vi "GF_SaveAgilentDataBinary.vi"(1 "Array":waveform(dbl)[][](array[waveform]), 2 "Base Path":path) -> (0 "File Write Errors":errorcluster[](array[cluster]))   [LabVIEW 2009]
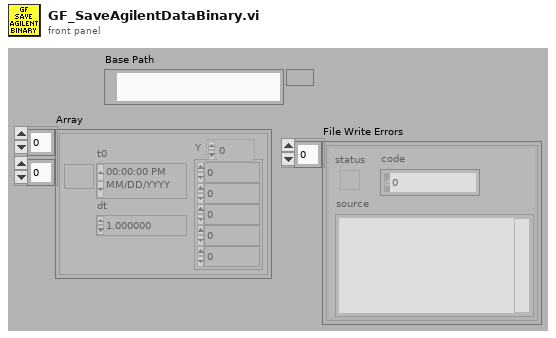
[diagram p1: front panel]
types:
  T1 = enum16{"big-endian, network order", "native, host order", "little-endian"}
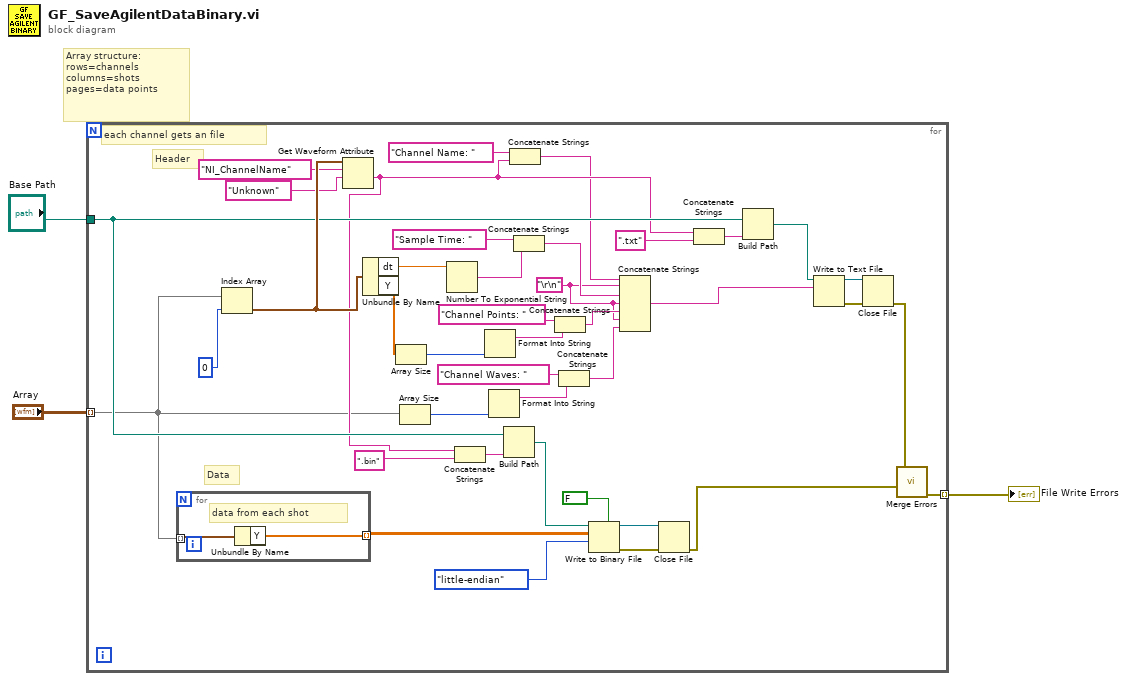
[diagram p0: block diagram]
diagram:
  # "Array structure:\nrows=channels\ncolumns=shots\npages=data points"
  n1 = for {
    tunnel: "Array" -> [w7] mode=indexing
    tunnel: "Base Path" -> [w26]
    tunnel: [w24] -> w1 mode=indexing
    w5 = "\r\n"
    # "Data"
    # "Header"
    # "each channel gets an file"
    n2 = for {
      tunnel: w7 -> [w45] mode=indexing
      tunnel: [w44] -> w31 mode=indexing
      # "data from each shot"
      n3 = Unbundle By Name(w45) -> ("Y"=w44:dbl[])
    }
    n4 = Index Array(array=w7, index=0) -> (element=w42:waveform(dbl))
    n5 = Get Waveform Attribute(5:"Unknown" ("name"), 6:"NI_ChannelName" ("name"), 7:w42) -> (1:w23:string)  [unwired: 1 in, 3 out]
    n6 = Unbundle By Name(w42) -> ("dt"=w39:dbl, "Y"=w14:dbl[])
    n7 = Array Size(array=w14) -> (size(s)=w12:i32)
    n8 = Array Size(array=w7) -> (size(s)=w8:i32)
    n9 = Number To Exponential String(number=w39) -> (E-format string=w38:string)  [unwired: 3 in]
    n10 = Concatenate Strings(w23, ".bin" ("string")) -> (w28:string)
    n11 = Format Into String(w12) -> (resulting string=w11:string)  [unwired: 3 in, 1 out]
    n12 = Format Into String(w8) -> (resulting string=w6:string)  [unwired: 3 in, 1 out]
    n13 = Build Path(base path=w26, name or relative path=w28) -> (appended path=w25:path)
    n14 = Concatenate Strings("Channel Name: " ("string"), w23) -> (w16:string)
    n15 = Concatenate Strings("Sample Time: " ("string"), w38) -> (w15:string)
    n16 = Concatenate Strings("Channel Points: " ("string"), w11) -> (w10:string)
    n17 = Concatenate Strings("Channel Waves: " ("string"), w6) -> (w4:string)
    n18 = Write to Binary File(file (use dialog)=w25, data=w31, 5:FALSE ("prepend array or string size? (T)"), 9:T1."little-endian" ("byte order (0:big-endian, network order)")) -> (refnum out=w22:refnum<file>, error out=w21:errorcluster)  [unwired: 2 in, 1 out]
    n19 = Concatenate Strings(w16, w5, w15, w5, w10, w5, w4) -> (w35:string)
    n20 = Close File(refnum=w22, error in=w21) -> (error out=w20:errorcluster)  [unwired: 1 out]
    n21 = Concatenate Strings(w23, ".txt" ("string")) -> (w33:string)
    n22 = Build Path(base path=w26, name or relative path=w33) -> (appended path=w32:path)
    n23 = Write to Text File(file (use dialog)=w32, text=w35) -> (refnum out=w19:refnum<file>, error out=w18:errorcluster)  [unwired: 2 in, 1 out]
    n24 = Close File(refnum=w19, error in=w18) -> (error out=w17:errorcluster)  [unwired: 1 out]
    n25 = call <vilib>:"Merge Errors.vi"("error in 3 (no error)"=w20, "error in 1 (no error)"=w17) -> ("error out"=w24:errorcluster)  [unwired: 5 in]
  }
  "File Write Errors" <- w1
